vi "Get Chamber Status-UTF-Setup.vi"   [LabVIEW 2018]
uses:
  Libraries/Thermal Chamber Response Simulator/Thermal Chamber Response Simulator.lvlib
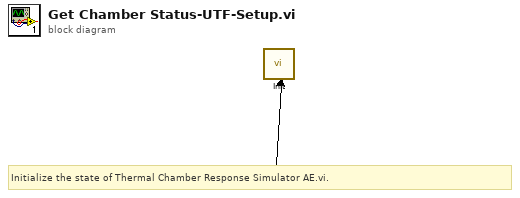
[diagram p0: block diagram]
diagram:
  # "Initialize the state of Thermal Chamber Response Simulator AE.vi."
  n1 = call "Init.vi"() -> ()  [unwired: 11 in, 1 out]
